vi "Housekeeping Management Core.vi"(11 "CIFPluginManager in":refnum<class "CIFPluginManager.lvclass">) -> (0 "error out":errorcluster)   [LabVIEW 2021, in "CIFPluginManager.lvclass"]
uses:
  CIFPluginManager.lvclass
  CIFPluginManager.lvclass/CIFPluginManager.ctl
  CIFUtilities/CIFLogs/Typedef/Message Type.ctl
  <vilib>/Utility/miscctls.llb/LVMapReplaceAction.ctl
  CIFUtilities/CIFLogs/CIFLogs.lvlib
  gRPC/CIF_Manager_Client_Wrapper/CIFManagerClientWrapper.lvlib
  <vilib>/CIF Foundation/CIF Utilities/Time/Time_CIF_U.lvlib
  CIFPluginLoader/gRPC/CIF_Plugin_Loader_Client_Wrapper/CIFPluginLoaderClientWrapper.lvlib
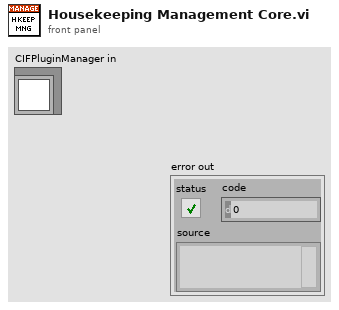
[diagram p1: front panel]
types:
  T1 = typedef "CIFLogs.lvlib/Message Type.ctl" = enum16{"Error", "Information", "Print Terminal", "Configuration"}
  T2 = typedef "LVMapReplaceAction.ctl" = enum32{"Modify Entry only if found", "Add or Modify Entry", "Delete Entry"}
  T3 = typedef "CIFPluginManager.lvclass/Loader Map.ctl" = map{string, T4}
  T4 = typedef "CIFPluginManager.lvclass/Loaders.ctl" = cluster{"Loader Type":T5, "grpc_port":i32, "pid":u32, "gRPC ID":T6, "Load Timestamp":i64, "Unloading":bool, "Ready for removal":bool, "Unload Timestamp":i64}
  T5 = typedef "CIFPluginManager.lvclass/Loader Type.ctl" = enum16{"LabVIEW"}
  T6 = typedef "grpc-lvsupport-release.lvlib/grpcId.ctl" = u64
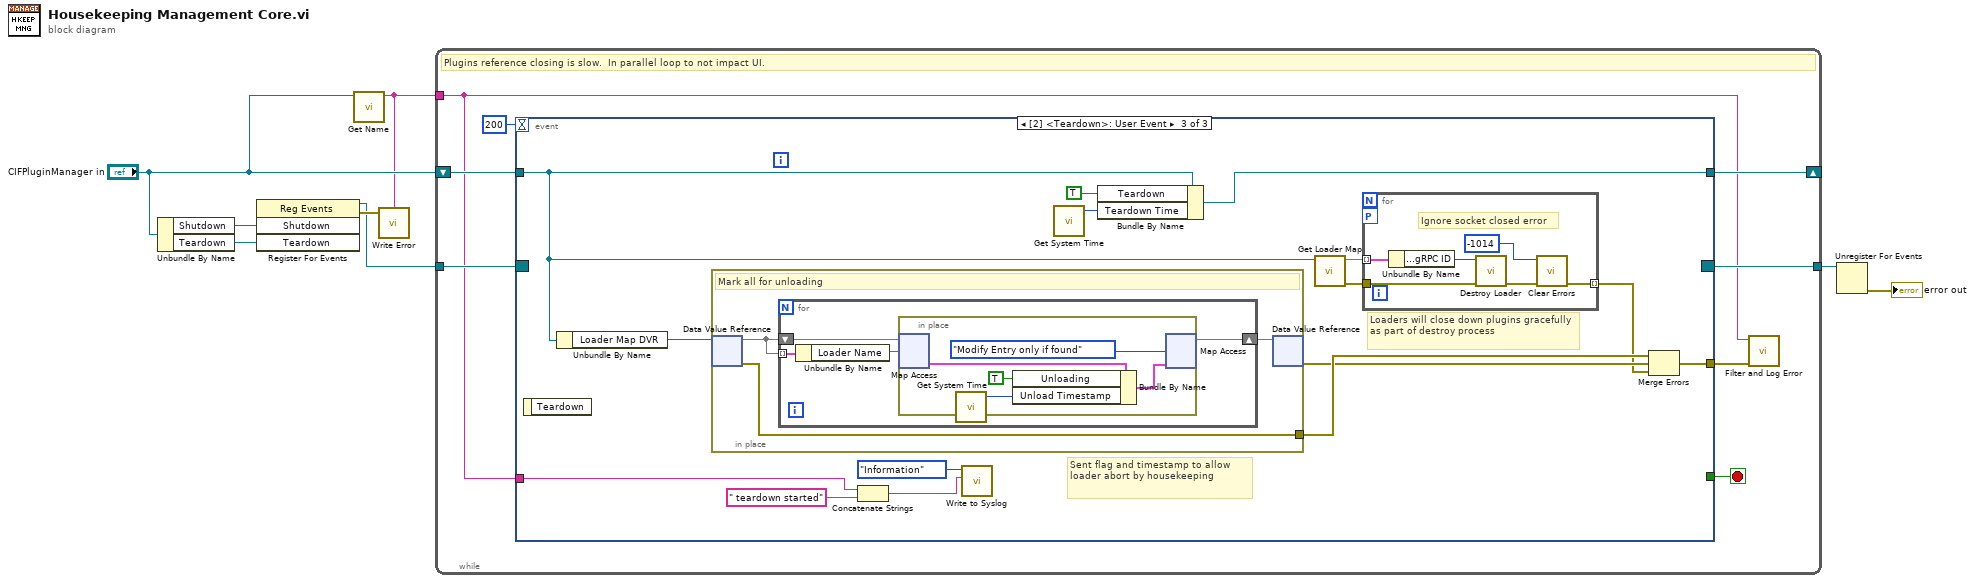
[diagram p0: block diagram]
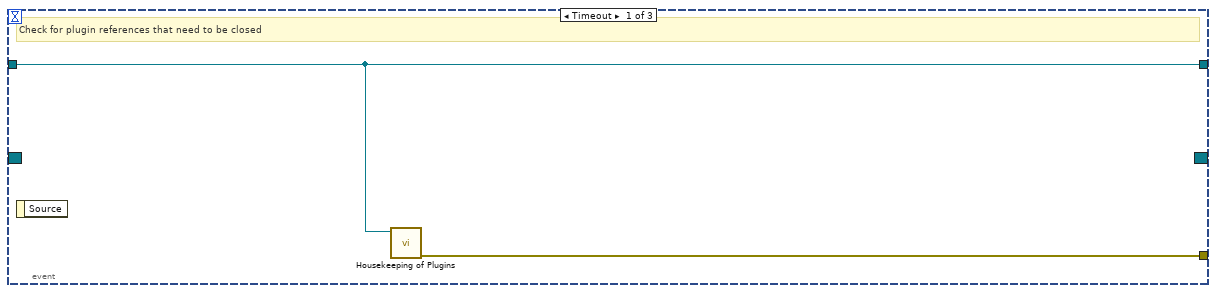
[diagram p2: hidden frame]
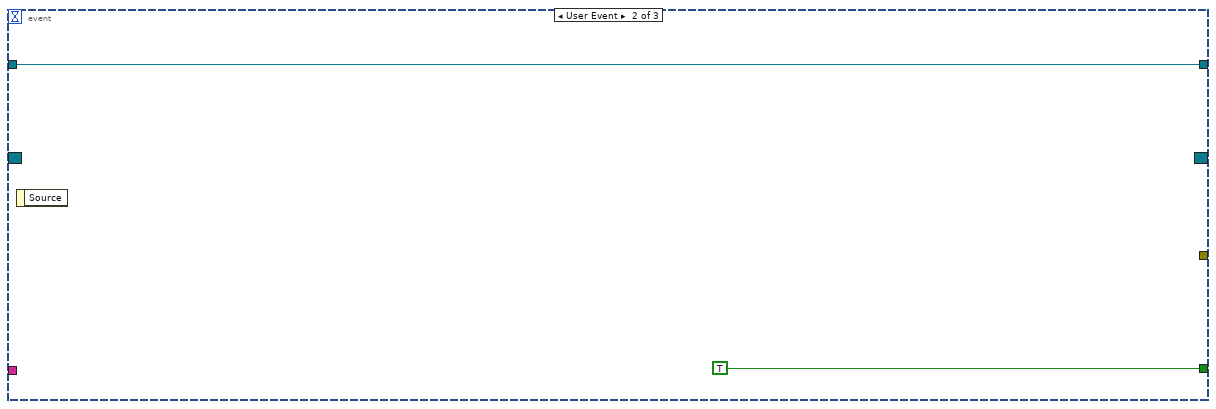
[diagram p3: hidden frame]
diagram:
  n1 = Unbundle By Name("CIFPluginManager in") -> ("Shutdown"=w4:refnum<user-event>, "Teardown"=w1:refnum<user-event>)
  n2 = register-events(w4, w1) -> (reference out=w5:refnum<event-registration>, error out=w6:errorcluster)  [unwired: 2 in]
  n3 = call "Get Name.vi"("CIFPluginManager in"="CIFPluginManager in") -> ("Name"=w2:string)  [unwired: 10 in]
  n4 = call "Write Error.vi"("error in (no error)"=w6, "Plugin Name"=w2) -> ()  [unwired: 2 in, 1 out]
  n5 = while {
    tunnel: w5 -> [w11]
    tunnel: [w13] -> w7
    tunnel: w2 -> [w9]
    shift-right: [w10] -> _
    shift-left: "CIFPluginManager in" -> [w16]
    stop <- w14 stop-if-true
    # "Plugins reference closing is slow.  In parallel loop to not impact UI."
    n6 = event shown="[2] <Teardown>: User Event" {
      selector: w11 -> [_ _ _]
      dyn-events: [_ _ _] -> w13
      timeout: 200 -> [_ _ _]
      tunnel: w16 -> [w17 w19 w24]
      tunnel: [_ TRUE _] -> w14
      tunnel: [w18 _ w21] -> w12
      tunnel: [w17 w19 w23] -> w10
      tunnel: w9 -> [_ _ w22]
      event Timeout {
        # "Check for plugin references that need to be closed"
        n7 = event-data() -> ()  [unwired: 1 in, 1 out]
        n8 = call "Housekeeping of Plugins.vi"("CIFPluginManager in"=w17) -> ("error out"=w18:errorcluster)  [unwired: 10 in]
      }
      event User Event {
        n9 = event-data() -> ()  [unwired: 1 in, 1 out]
      }
      event User Event {
        # "Loaders will close down plugins gracefully as part of destroy process"
        # "Sent flag and timestamp to allow loader abort by housekeeping"
        n10 = event-data() -> ()  [unwired: 1 in, 1 out]
        n11 = Unbundle By Name(w24) -> ("Loader Map DVR"=w35:refnum<data-value>)
        n12 = in-place {
          in-place-border: [w42] -> w32
          # "Mark all for unloading"
          n13 = in-place-dvr #1(w35) -> (w44:T3, w42:errorcluster)
          n14 = for {
            tunnel: w44 -> [w46] mode=indexing
            shift-right: [w47] -> w43
            shift-left: w44 -> [w48]
            n15 = Unbundle By Name(w46) -> ("Loader Name"=w45:string)
            n16 = in-place {
              n17 = in-place-map #2(w48, w45) -> (w50:T4)  [unwired: 1 in, 1 out]
              n18 = call <vilib>:"Get System Time.vi"() -> ("Time (ns)"=w51:i64)  [unwired: 5 in]
              n19 = Bundle By Name(cluster=w50, "Unloading"=TRUE, "Unload Timestamp"=w51) -> (w49:T4)
              n20 = in-place-map #2(w49, LVMapReplaceAction."Modify Entry only if found" ("action")) -> (w47:T3)  [unwired: 2 out]
            }
          }
          n21 = in-place-dvr #1(w43) -> (w31:errorcluster)  [unwired: 1 out]
        }
        n22 = Concatenate Strings(w22, " teardown started" ("message")) -> (w26:string)
        n23 = call "Write to Syslog.vi"("message"=w26, "CIF Message Type"=Message_Type."Information") -> ()  [unwired: 9 in, 1 out]
        n24 = call <vilib>:"Get System Time.vi"() -> ("Time (ns)"=w29:i64)  [unwired: 5 in]
        n25 = Bundle By Name(cluster=w24, "Teardown"=TRUE ("Unloading"), "Teardown Time"=w29) -> (w23:refnum<class "CIFPluginManager.lvclass">)
        n26 = call "Get Loader Map.vi"("CIFPluginManager in"=w24) -> ("error out"=w33:errorcluster, "Loader Map"=w34:T3)  [unwired: 9 in]
        n27 = for {
          tunnel: w33 -> [w38]
          tunnel: w34 -> [w41] mode=indexing
          workers-P: _ -> [_]
          tunnel: [w40] -> w30 mode=indexing
          # "Ignore socket closed error"
          n28 = Unbundle By Name(w41) -> ("Loaders.gRPC ID"=w37:T6)
          n29 = call "Destroy Loader.vi"("error in"=w38, "gRPC ID in"=w37) -> ("error out"=w36:errorcluster)  [unwired: 8 in, 1 out]
          n30 = call <vilib>:"Clear Errors.vi"("error in (no error)"=w36, "specific error code to clear (0: all)"=-1014) -> ("error out"=w40:errorcluster)  [unwired: 4 in, 1 out]
        }
        n31 = Merge Errors(w32, w31, w30) -> (w21:errorcluster)
      }
    }
    n32 = call "Filter and Log Error.vi"("error In"=w12, "Name"=w9) -> ()  [unwired: 10 in]
  }
  n33 = Unregister For Events(event registration refnum=w7) -> (error out=→"error out":errorcluster)  [unwired: 1 in]
